vi "Check CS Lines vs Channels.vi"(8 "error in":errorcluster, 11 "Bus Info":T1[](array[typedef])) -> (0 "error out":errorcluster)   [LabVIEW 2014, in "Initialization and IO Node Scripting.lvlib"]
uses:
  Initialization and IO Node Scripting.lvlib
  State Machine/Controls/Device Information.ctl
  State Machine/Controls/Pin Information.ctl
  State Machine/Controls/Bus Information.ctl
  <vilib>/LabVIEW Icon API/API_Text.ctl
  <vilib>/LabVIEW Icon API/LabVIEW Icon API.lvlib
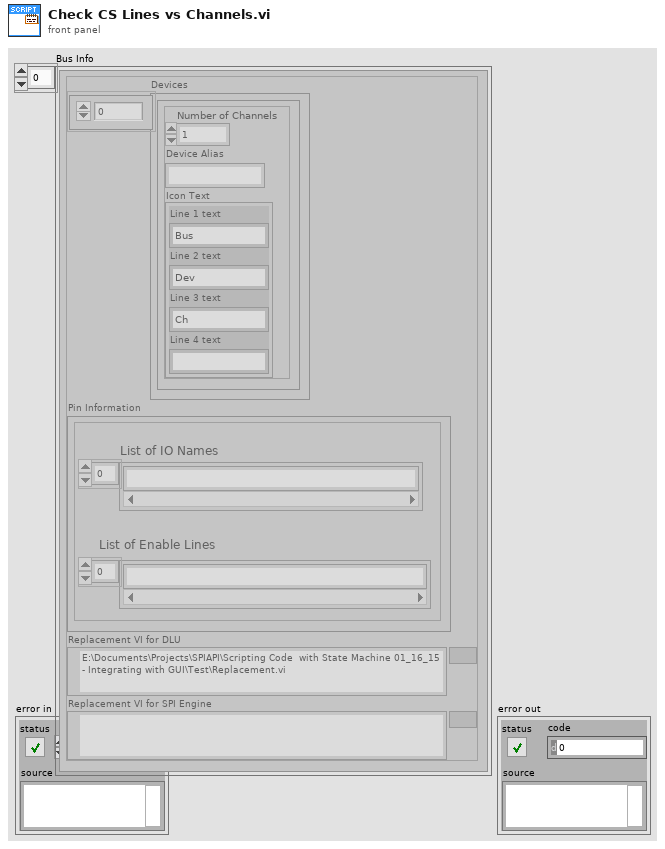
[diagram p1: front panel]
types:
  T1 = typedef "Initialization and IO Node Scripting.lvlib/Bus Information.ctl" = cluster{"Devices":T2[], "Pin Information":T4, "Replacement VI for DLU":path, "Replacement VI for SPI Engine":path}
  T2 = typedef "Device Information.ctl" = cluster{"Number of Channels":i32, "Device Alias":string, "Icon Text":T3}
  T3 = typedef "LabVIEW Icon API.lvlib/API_Text.ctl" = cluster{"Line 1 text":string, "Line 2 text":string, "Line 3 text":string, "Line 4 text":string}
  T4 = typedef "Pin Information.ctl" = cluster{"List of IO Names":string[], "List of Enable Lines":string[]}
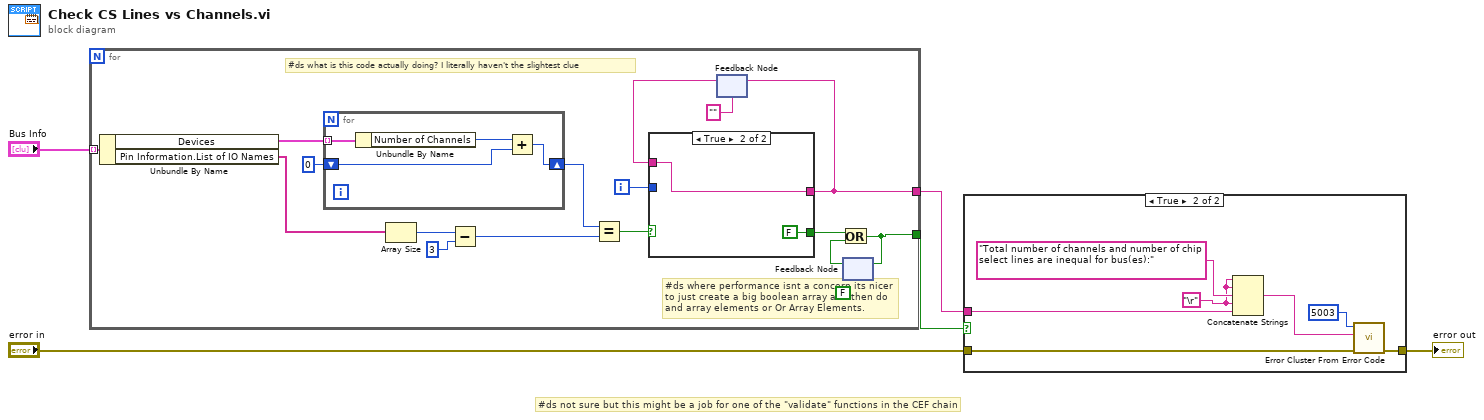
[diagram p0: block diagram]
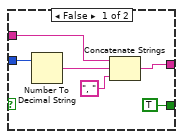
[diagram p3: hidden frame]
diagram:
  # "#ds not sure but this might be a job for one of the \"validate\" functions in the CEF chain"
  n1 = for {
    tunnel: "Bus Info" -> [w22] mode=indexing
    tunnel: [w10] -> w4
    tunnel: [w6] -> w5
    i -> [w14]
    # "#ds where performance isnt a concern its nicer \nto just create a big boolean array and then do\nand array elements or Or Array Elements."
    # "#ds what is this code actually doing? I literally haven't the slightest clue"
    n2 = Unbundle By Name(w22) -> ("Devices"=w21:T2[], "Pin Information.List of IO Names"=w20:string[])
    n3 = for {
      tunnel: w21 -> [w34] mode=indexing
      shift-right: [w33] -> w16
      shift-left: 0 -> [w31]
      n4 = Unbundle By Name(w34) -> ("Number of Channels"=w32:i32)
      n5 = Add(x=w32, y=w31) -> (x+y=w33:i32)
    }
    n6 = Array Size(array=w20) -> (size(s)=w19:i32)
    n7 = Subtract(x=w19, y=3) -> (x-y=w15:i32)
    n8 = Equal?(x=w16, y=w15) -> (x = y?=w13:bool)
    n9 = feedback #1("") -> (w12:string)
    n10 = case shown="True" w13 {
      tunnel: w14 -> [w28 _]
      tunnel: [w27 w30] -> w10
      tunnel: w12 -> [w25 w30]
      tunnel: [TRUE FALSE] -> w9
      frame False {
        n11 = Number To Decimal String(number=w28) -> (decimal integer string=w26:string)  [unwired: 1 in]
        n12 = Concatenate Strings(w25, w26, ", " ("string")) -> (w27:string)
      }
      frame True {
      }
    }
    n13 = feedback-in #1(w10) -> ()
    n14 = feedback #2(FALSE) -> (w7:bool)
    n15 = Or(x=w9, y=w7) -> (x .or. y?=w6:bool)
    n16 = feedback-in #2(w6) -> ()
  }
  n17 = case shown="True" w5 {
    tunnel: "error in" -> [w35 w42]
    tunnel: [w35 w40] -> w3
    tunnel: w4 -> [_ w37]
    frame False {
    }
    frame True {
      w36 = "\r"
      n18 = Concatenate Strings(w36, w36, "Total number of channels and number of chip select lines are inequal for bus(es):" ("error message (\"\")"), w36, w37) -> (w38:string)
      n19 = call <vilib>:"Error Cluster From Error Code.vi"("error in (no error)"=w42, "error message (\"\")"=w38, "error code (0)"=5003) -> ("error out"=w40:errorcluster)  [unwired: 6 in]
    }
  }
  "error out" <- w3
